vi "MtAtElectrometer_flushSamplesEvent_errorCode.vi"(8 "error in (no error)":errorcluster) -> (0 "error out":errorcluster, 3 "function return":i32)   [LabVIEW 2016, in "SALLV_MtAtElectrometer.lvlib"]
doc: "int MtAtElectrometer_shm_flushSamplesEvent_errorCodeLV();"
uses:
  SALLV_MtAtElectrometer.lvlib
  ts_sal/test/MtAtElectrometer/labview/SALLV_MtAtElectrometer.so
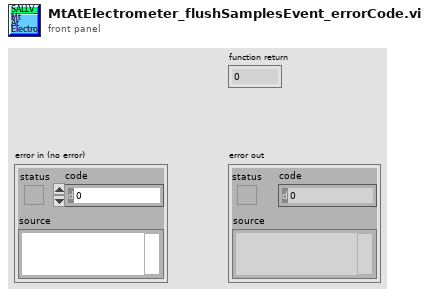
[diagram p1: front panel]
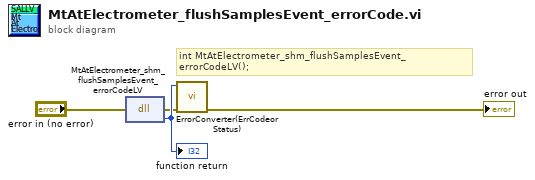
[diagram p0: block diagram]
diagram:
  # "int MtAtElectrometer_shm_flushSamplesEvent_errorCodeLV();"
  n1 = dll-call lib="home/andres/ts_sal/test/MtAtElectrometer/labview/SALLV_MtAtElectrometer.*" fn="MtAtElectrometer_shm_flushSamplesEvent_errorCodeLV"(error in="error in (no error)") -> (error out=w2:errorcluster, w4:i32)  [unwired: 2 in, 1 out]
  "function return" <- w4
  n2 = call "ErrorConverter(ErrCodeorStatus).vi"("error in (no error)"=w2, "error code"=w4) -> ("error out"=→"error out":errorcluster)  [unwired: 9 in]
